vi "_Write.vi"(7 "File Size Limit (Bytes)":i64, 8 "Error In":errorcluster, 10 "Messages":T1[](array[typedef]), 11 "Log In":refnum<file>) -> (0 "Error Out":errorcluster, 3 "Log Out":refnum<file>)   [LabVIEW 2014, in "LV-Logger.lvlib"]
uses:
  LV-Logger.lvlib
  Public/Controls/Message.ctl
  Public/Controls/Tag.ctl
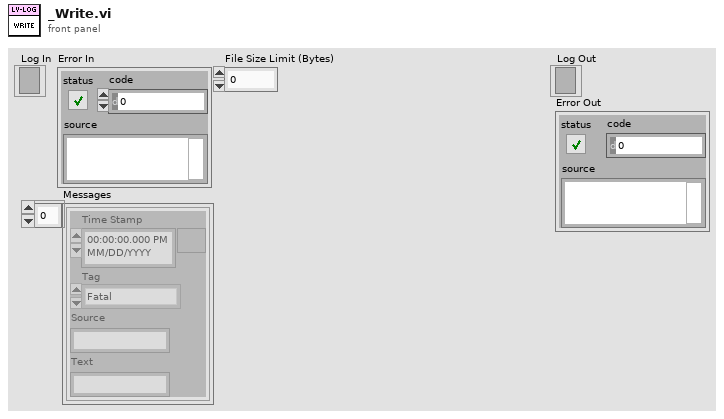
[diagram p1: front panel]
types:
  T1 = typedef "LV-Logger.lvlib/Message.ctl" = cluster{"Time Stamp":timestamp, "Tag":T2, "Source":string, "Text":string}
  T2 = typedef "LV-Logger.lvlib/Tag.ctl" = enum16{"Fatal", "Error", "Warn", "Info", "Debug", "Trace"}
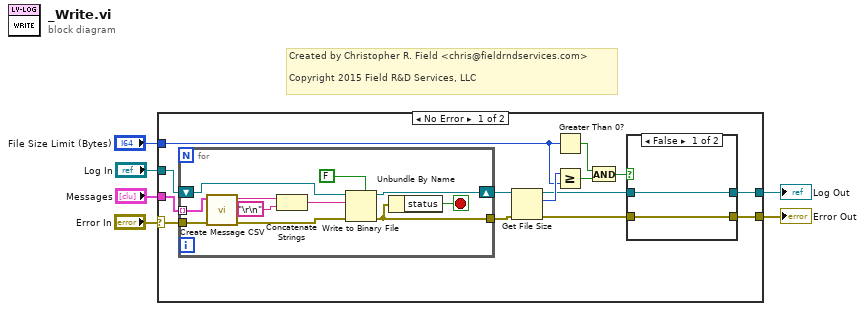
[diagram p0: block diagram]
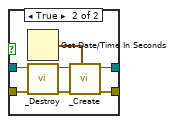
[diagram p2: hidden frame]
diagram:
  # "Created by Christopher R. Field <chris@fieldrndservices.com>\n\nCopyright 2015 Field R&D Services, LLC"
  n1 = case shown="No Error" "Error In" {
    selector: "Error In" -> [w19 w41]
    tunnel: "Log In" -> [w20 w42]
    tunnel: "Messages" -> [w18 _]
    tunnel: [w8 w42] -> w3
    tunnel: [w7 w41] -> w2
    tunnel: "File Size Limit (Bytes)" -> [w9 _]
    frame No Error {
      n2 = for {
        tunnel: w19 -> [w36]
        tunnel: w18 -> [w33] mode=indexing
        shift-right: [w31] -> w11
        shift-left: w20 -> [w38]
        tunnel: [w30] -> w10
        stop <- w32 stop-if-true
        n3 = call "Create Message CSV.vi"("Error In"=w36, "Message"=w33) -> ("Error Out"=w35:errorcluster, "CSV"=w34:string)  [unwired: 8 in]
        n4 = Concatenate Strings(w34, "\r\n") -> (w39:string)
        n5 = Write to Binary File(file (use dialog)=w38, data=w39, error in=w35, 5:FALSE ("prepend array or string size? (T)")) -> (refnum out=w31:refnum<file>, error out=w30:errorcluster)  [unwired: 2 in, 1 out]
        n6 = Unbundle By Name(w30) -> ("status"=w32:bool)
      }
      n7 = Get File Size(file=w11, error in=w10) -> (refnum out=w13:refnum<file>, size (in bytes)=w15:i64, 0:w12:errorcluster)
      n8 = Greater Than 0?(x=w9) -> (x > 0?=w16:bool)
      n9 = Greater Or Equal?(x=w15, y=w9) -> (x >= y?=w17:bool)
      n10 = And(x=w16, y=w17) -> (x .and. y?=w14:bool)
      n11 = case shown="False" w14 {
        tunnel: [w22 w28] -> w8
        tunnel: [w21 w27] -> w7
        tunnel: w13 -> [w22 w26]
        tunnel: w12 -> [w21 w25]
        frame False {
        }
        frame True {
          n12 = Get Date/Time In Seconds() -> (seconds since 1Jan1904=w29:timestamp)
          n13 = call "_Destroy.vi"("Error In"=w25, "Log In"=w26) -> ("Error Out"=w23:errorcluster, "Base Log Folder"=w24:path)  [unwired: 8 in]
          n14 = call "_Create.vi"("Start Time Stamp"=w29, "Error In"=w23, "Base Log Folder"=w24) -> ("Error Out"=w27:errorcluster, "Log Out"=w28:refnum<file>)  [unwired: 7 in]
        }
      }
    }
    frame Error {
    }
  }
  "Log Out" <- w3
  "Error Out" <- w2
